vi "Untitled 1 (SubVI).vi"(11 "Image Out":T1 {"Dialogs" format="%.0b"}) -> (1 "Cb":dbl[][](array[numeric]), 2 "Cr":dbl[][](array[numeric]), 3 "result":dbl[][](array[numeric]))   [LabVIEW 2012]
uses:
  <userlib>/ImageProcessing/QTLIB_2595_LV86/QT_Image.ctl
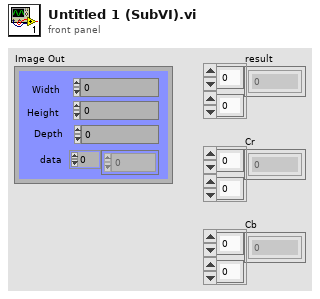
[diagram p1: front panel]
types:
  T1 = typedef "QT_Image.ctl" = cluster{"Width":i32, "Height":i32, "Depth":i32, "data":u8[], "Compressed data":u8[], "Color table":u32[], "Duration":i32, "Options":i32, "Timestamp":i32, "ID":i32, "Reserved":i32, "Dialogs":u32}
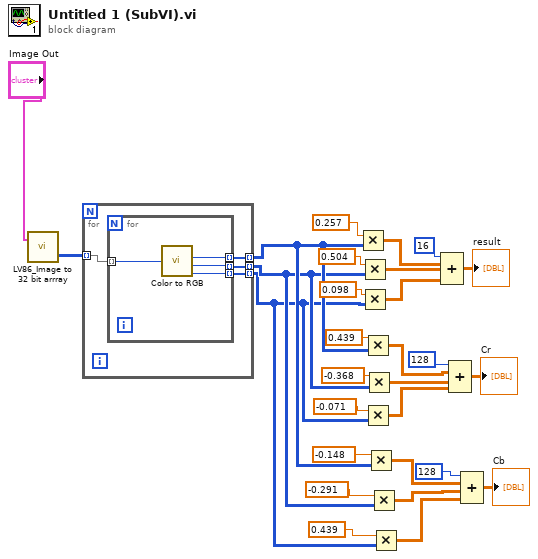
[diagram p0: block diagram]
diagram:
  n1 = call <userlib>:"LV86_Image to 32 bit arrray.vi"("Image In"="Image Out") -> ("Intensity Graph"=w27:u32[][])  [unwired: 1 in, 1 out]
  n2 = for {
    tunnel: w27 -> [w33] mode=indexing
    tunnel: [w32] -> w26 mode=indexing
    tunnel: [w31] -> w25 mode=indexing
    tunnel: [w30] -> w24 mode=indexing
    n3 = for {
      tunnel: w33 -> [w37] mode=indexing
      tunnel: [w36] -> w32 mode=indexing
      tunnel: [w35] -> w31 mode=indexing
      tunnel: [w34] -> w30 mode=indexing
      n4 = call <vilib>:"Color to RGB.vi"("Color"=w37) -> ("R"=w36:u8, "G"=w35:u8, "B"=w34:u8)  [unwired: 1 out]
    }
  }
  n5 = Multiply(x=0.257, y=w26) -> (x*y=w20:dbl[][])
  n6 = Multiply(x=0.504, y=w25) -> (x*y=w19:dbl[][])
  n7 = Multiply(x=0.098, y=w24) -> (x*y=w18:dbl[][])
  n8 = Multiply(x=0.439, y=w26) -> (x*y=w10:dbl[][])
  n9 = Multiply(x=-0.071, y=w24) -> (x*y=w8:dbl[][])
  n10 = Multiply(x=-0.368, y=w25) -> (x*y=w9:dbl[][])
  n11 = Multiply(x=-0.148, y=w26) -> (x*y=w5:dbl[][])
  n12 = Multiply(x=-0.291, y=w25) -> (x*y=w4:dbl[][])
  n13 = Multiply(x=0.439, y=w24) -> (x*y=w3:dbl[][])
  n14 = Compound Arithmetic op=ADD(16, w20, w19, w18) -> (→"result":dbl[][])
  n15 = Compound Arithmetic op=ADD(128, w10, w9, w8) -> (→"Cr":dbl[][])
  n16 = Compound Arithmetic op=ADD(128, w5, w4, w3) -> (→"Cb":dbl[][])
